vi "Serial Control.vi"(0 "VISA resource name":refnum<visa-resource-name>, 1 "Reset":bool, 2 "Buffer_in":string, 3 "Frequency Write":dbl, 4 "write buffer":string) -> (5 "error IO":errorcluster, 6 "Buffer_out":string, 7 "Write Count":u16)   [LabVIEW 2022 SP3]
uses:
  <vilib>/Instr/_visa.llb/VISA Configure Serial Port (Instr).vi
panel:
  in  "Sync  End":u8=109
  in  "Sync Begin":u8=146
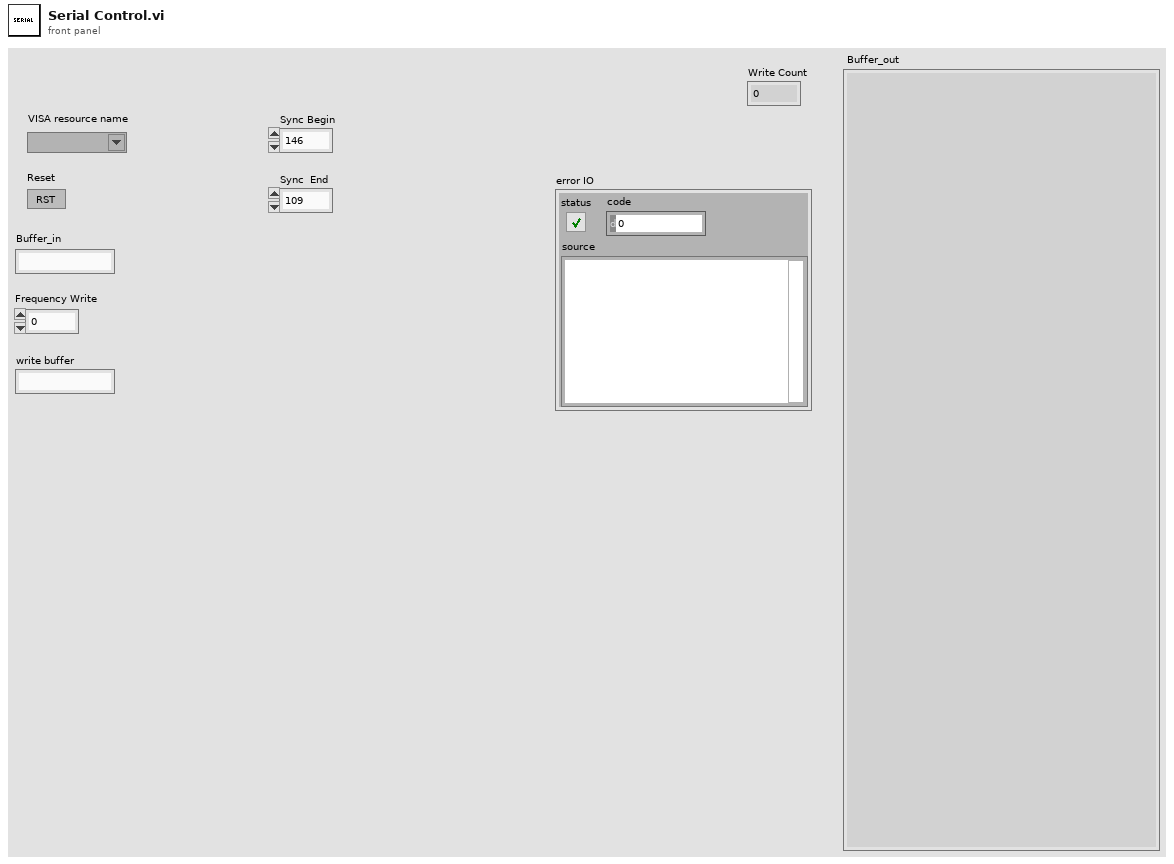
[diagram p1: front panel]
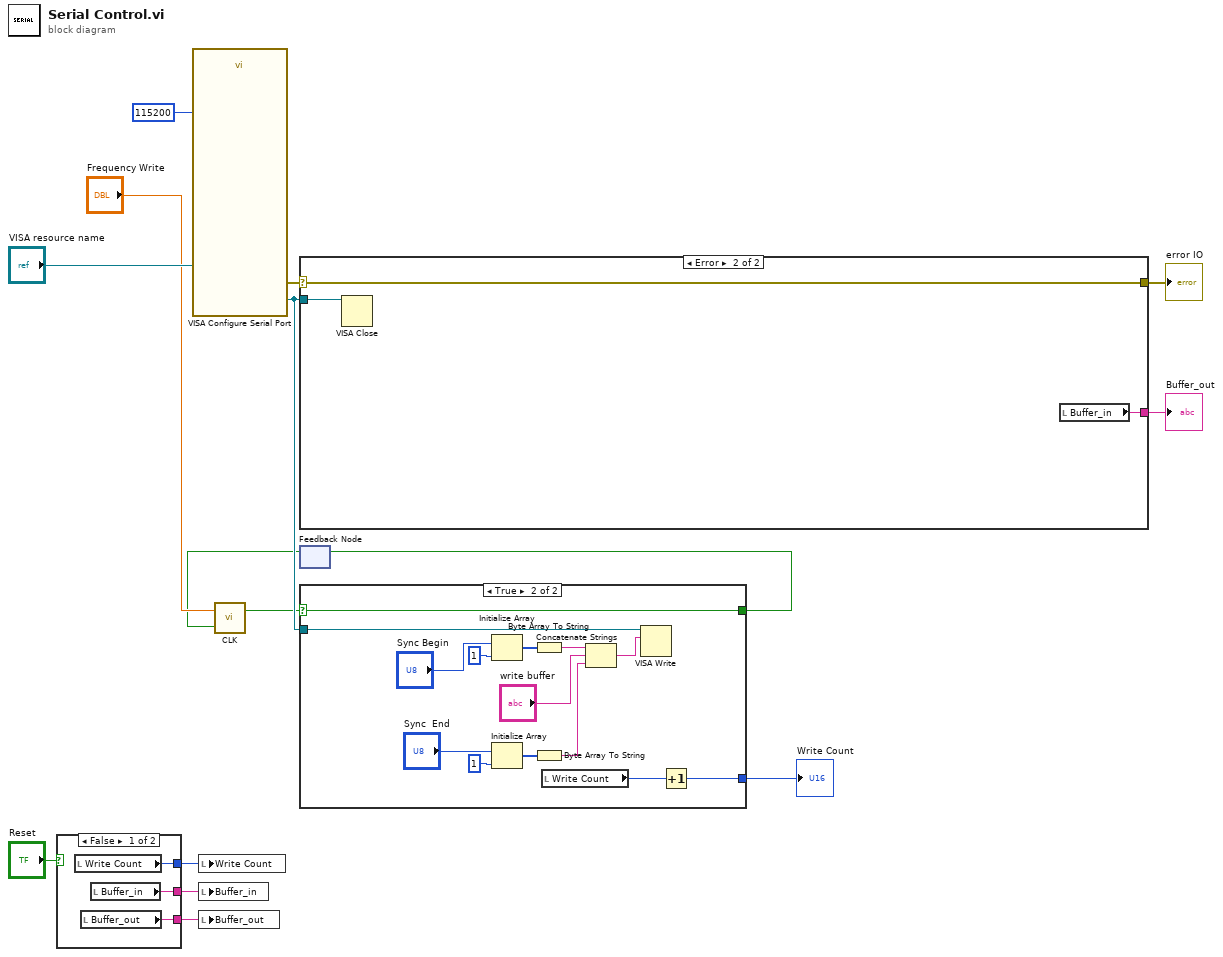
[diagram p0: block diagram]
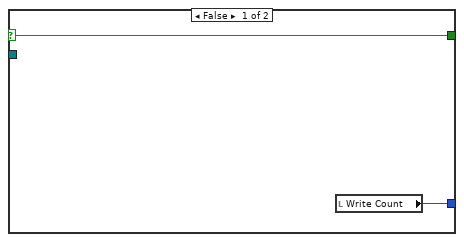
[diagram p2: hidden frame]
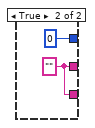
[diagram p3: hidden frame]
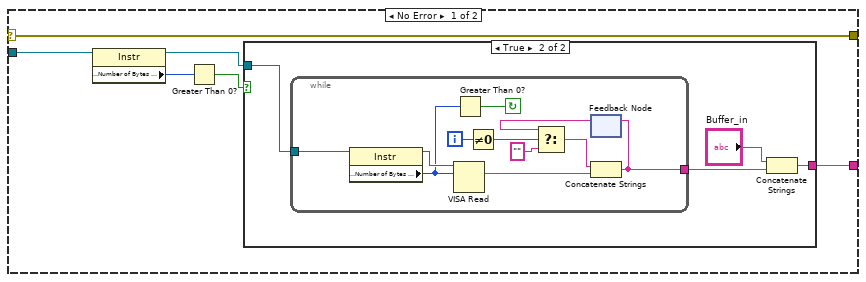
[diagram p4: hidden frame]
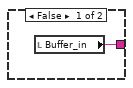
[diagram p5: hidden frame]
diagram:
  n1 = case shown="False" "Reset" {
    tunnel: [w17 w20] -> w8
    tunnel: [w18 w20] -> w7
    tunnel: [w16 u16 0 ("Write Count")] -> w6
    frame False {
      n2 = local read "Write Count"() -> (w16:u16)
      n3 = local read "Buffer_out"() -> (w18:string)
      n4 = local read "Buffer_in"() -> (w17:string)
    }
    frame True {
      w20 = ""
    }
  }
  n5 = call-poly "VISA Configure Serial Port"("VISA resource name"="VISA resource name", "baud rate (9600)"=u32 115200) -> ("VISA resource name out"=w5:refnum<visa-resource-name>, "error out"=w13:errorcluster)  [unwired: 12 in]
  n6 = local write "Write Count"(w6) -> ()
  n7 = local write "Buffer_in"(w8) -> ()
  n8 = local write "Buffer_out"(w7) -> ()
  n9 = case shown="No Error" w13 {
    selector: w13 -> [w21 w44]
    tunnel: w5 -> [w26 w43]
    tunnel: [w22 w45] -> w12
    tunnel: [w21 w44] -> w10
    frame No Error {
      n10 = property class="Instr"(reference=w26) -> (reference out=w24:refnum<visa-resource-name>, "Serial Settings:Number of Bytes at Serial Port"=w25:u32)  [unwired: 1 in, 1 out]
      n11 = Greater Than 0?(x=w25) -> (x > 0?=w23:bool)
      n12 = case shown="True" w23 {
        tunnel: w24 -> [_ w31]
        tunnel: [w27 w28] -> w22
        frame False {
          n13 = local read "Buffer_in"() -> (w27:string)
        }
        frame True {
          n14 = while {
            tunnel: w31 -> [w36]
            tunnel: [w32] -> w30
            i -> [w37]
            stop <- w33 continue-if-true
            n15 = property class="Instr"(reference=w36) -> (reference out=w35:refnum<visa-resource-name>, "Serial Settings:Number of Bytes at Serial Port"=w34:u32)  [unwired: 1 in, 1 out]
            n16 = VISA Read(VISA resource name=w35, byte count=w34) -> (read buffer=w40:string)  [unwired: 1 in, 3 out]
            n17 = Greater Than 0?(x=w34) -> (x > 0?=w33:bool)
            n18 = Not Equal To 0?(x=w37) -> (x != 0?=w38:bool)
            n19 = feedback #1() -> (w41:string)  [unwired: 1 in]
            n20 = Select(t=w41, s=w38, f="") -> (s? t:f=w42:string)
            n21 = Concatenate Strings(w42, w40) -> (w32:string)
            n22 = feedback-in #1(w32) -> ()
          }
          n23 = Concatenate Strings("Buffer_in", w30) -> (w28:string)
        }
      }
    }
    frame Error {
      n24 = VISA Close(VISA resource name=w43) -> ()  [unwired: 1 in, 1 out]
      n25 = local read "Buffer_in"() -> (w45:string)
    }
  }
  "Buffer_out" <- w12
  "error IO" <- w10
  n26 = feedback #2() -> (w1:bool)  [unwired: 1 in]
  n27 = call "CLK.vi"("Reset"=w1, "Frequency [Hz]"="Frequency Write") -> ("Output"=w4:bool)  [unwired: 1 out]
  n28 = case shown="True" w4 {
    selector: w4 -> [w47 w57]
    tunnel: [w47 w57] -> w2
    tunnel: [w46 w60] -> w9
    tunnel: w5 -> [_ w56]
    frame False {
      n29 = local read "Write Count"() -> (w46:u16)
    }
    frame True {
      n30 = Initialize Array("Sync Begin", 1 ("dimension size")) -> (w54:u8[])
      n31 = Initialize Array("Sync  End", 1 ("dimension size")) -> (w50:u8[])
      n32 = Byte Array To String(unsigned byte array=w54) -> (string=w52:string)
      n33 = Byte Array To String(unsigned byte array=w50) -> (string=w49:string)
      n34 = local read "Write Count"() -> (w61:u16)
      n35 = Concatenate Strings(w52, "write buffer", w49) -> (w58:string)
      n36 = VISA Write(VISA resource name=w56, write buffer=w58) -> ()  [unwired: 1 in, 3 out]
      n37 = Increment(x=w61) -> (x+1=w60:u16)
    }
  }
  "Write Count" <- w9
  n38 = feedback-in #2(w2) -> ()
